vi "TestExec.Factory Logix UUT Step Check, Use DB Stored Procedure.vi"(8 "error in (no error)":errorcluster, 9 "SN":string="SB74900285", 11 "UDL File":path=path "c:/MTE/FactoryLogix/FactoryLogix Connection.udl") -> (3 "Results":string[][](table))   [LabVIEW 2018]
doc: "This VI calls stored procedures in SQL Server using the LabVIEW Database Connectivity Toolset. The VI uses two methods to call the built-in stored procedure sp_helpuser -- one method uses parameters and the other does not."
uses:
  <vilib>/addons/database/Connection.llb/DB Tools Open Connec (Path).vi
  <vilib>/addons/database/Connection.llb/Conn Execute.vi
  <vilib>/addons/database/Recordset.llb/Rec Fetch Recordset Data (R).vi
  <vilib>/addons/database/Recordset.llb/Rec Destroy - Connection.vi
  <vilib>/addons/database/_DB Variant To Data/Database Variant To Data.xnode
  <vilib>/addons/database/NI_Database_API.lvlib
panel:
  out "error out":errorcluster
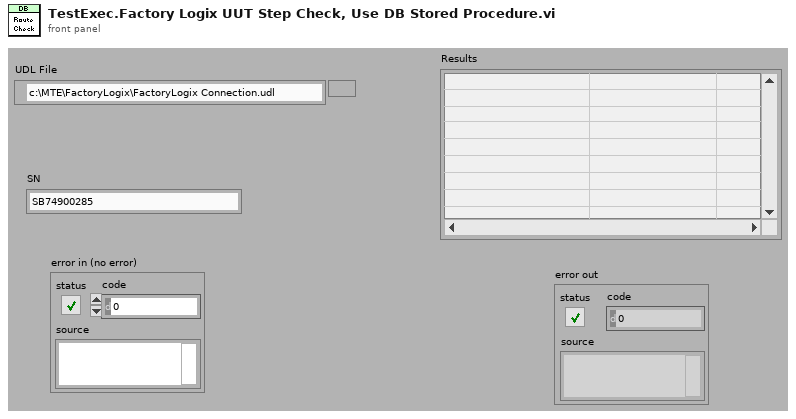
[diagram p1: front panel]
types:
  T1 = typedef "NI_Database_API.lvlib/Conn ObjectReference.ctl" = refnum<k1>
  T2 = typedef "NI_Database_API.lvlib/Rec ObjectReference.ctl" = refnum<k1>
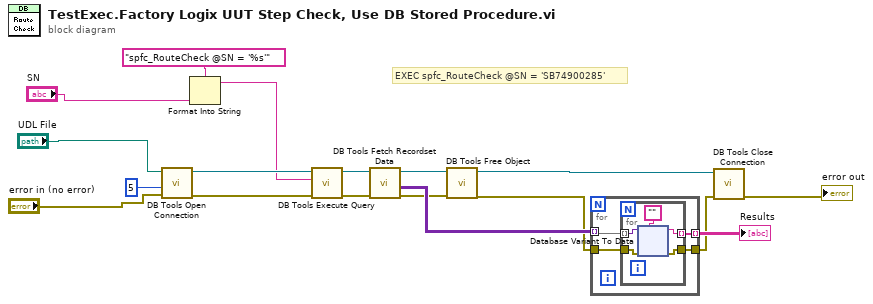
[diagram p0: block diagram]
diagram:
  # "EXEC spfc_RouteCheck @SN = 'SB74900285'"
  n1 = call-poly <vilib>:"DB Tools Open Connection.vi"("error in (no error)"="error in (no error)", "connection timeout (15)"=5, "connection information"="UDL File") -> ("error out"=w18:errorcluster, "connection reference"=w17:T1)  [unwired: 5 in]
  n2 = Format Into String(format string="spfc_RouteCheck @SN = '%s'", "SN") -> (resulting string=w3:string)  [unwired: 2 in, 1 out]
  n3 = call-poly <vilib>:"DB Tools Execute Query.vi"("error in (no error)"=w18, "SQL query"=w3, "connection reference"=w17) -> ("error out"=w7:errorcluster, "recordset reference"=w8:T2)  [unwired: 5 in]
  n4 = call-poly <vilib>:"DB Tools Fetch Recordset Data.vi"("error in (no error)"=w7, "recordset reference"=w8) -> ("error out"=w5:errorcluster, "recordset data"=w15:variant[][], "recordset reference out"=w6:T2)  [unwired: 3 in]
  n5 = call-poly <vilib>:"DB Tools Free Object.vi"("error in (no error)"=w5, "recordset reference"=w6) -> ("error out"=w14:errorcluster, "connection reference"=w12:T1)  [unwired: 8 in]
  n6 = for {
    tunnel: [w22] -> w16 mode=indexing
    tunnel: w15 -> [w21] mode=indexing
    tunnel: w14 -> [w20]
    tunnel: [w19] -> w13
    n7 = for {
      tunnel: [w26] -> w22 mode=indexing
      tunnel: w21 -> [w25] mode=indexing
      tunnel: w20 -> [w24]
      tunnel: [w23] -> w19
      n8 = xnode "Database Variant To Data"("database variant"=w25, "error in (no error)"=w24, "type"="") -> ("data"=w26:string, "error out"=w23:errorcluster)
    }
  }
  "Results" <- w16
  n9 = call <vilib>:"DB Tools Close Connection.vi"("error in (no error)"=w13, "connection reference"=w12) -> ("error out"=→"error out":errorcluster)  [unwired: 5 in]
